vi "SPI Flash Read Fast.vi"(6 "ReadLen":i32, 7 "pReadData":u8[](array[numeric])=array[4097 elements], 9 "StartAddr":i32, 10 "SPIIndex":i32, 11 "DevHandle":i32) -> (3 "function return":i32, 5 "pReadData out":u8[](array[numeric]))   [LabVIEW 2010, in "usb2spi.lvlib"]
doc: "int WINAPI SPI_FlashReadFast(int DevHandle,int SPIIndex,int StartAddr,unsigned char *pReadData,int ReadLen);"
uses:
  usb2spi.lvlib
  USB2XXX.dll
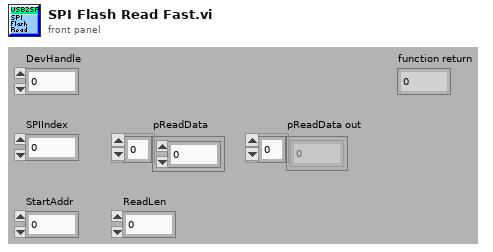
[diagram p1: front panel]
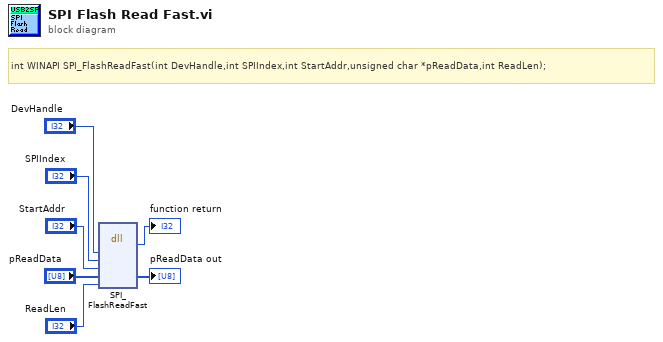
[diagram p0: block diagram]
diagram:
  # "int WINAPI SPI_FlashReadFast(int DevHandle,int SPIIndex,int StartAddr,unsigned char *pReadData,int ReadLen);"
  n1 = dll-call lib="G:/OtherWork/USB2XXX_Example/trunk/Labview/PublicFiles/USB2XXX.*" fn="SPI_FlashReadFast"("DevHandle"="DevHandle", "SPIIndex"="SPIIndex", "StartAddr"="StartAddr", "pReadData"="pReadData", "ReadLen"="ReadLen") -> (→"function return":i32, "pReadData"=→"pReadData out":u8[])  [unwired: 7 in, 2 out]
